vi "LVObject to JSON - JSON Array - Is Wrapped in Object.vi"() -> ()   [LabVIEW 2017, in "JSON Serializable Serializer Tests.lvlib"]
uses:
  JSON Serializable Serializer Tests.lvlib
  JSON Serializable Serializer/JSON Serializable Serializer.lvclass
  <vilib>/addons/_JKI Toolkits/Caraya/classes/Assert/Assert Equal Value_Variant.vi
  <vilib>/addons/_JKI Toolkits/Caraya/classes/Test/Test.lvclass
  <vilib>/addons/_JKI Toolkits/Caraya/classes/Assert/Assert.lvclass
  Mock JSON Serializable/Mock JSON Serializable.lvclass
panel:
  out "error out":errorcluster
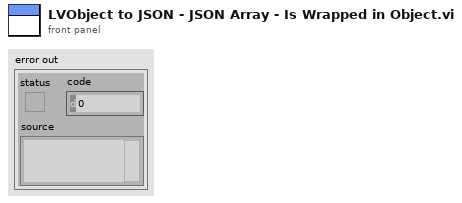
[diagram p1: front panel]
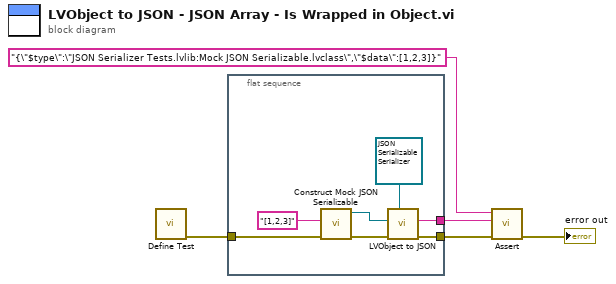
[diagram p0: block diagram]
diagram:
  n1 = call <vilib>:"Define Test.vi"() -> ("error out"=w4:errorcluster)  [unwired: 11 in]
  n2 = flat-sequence {
    tunnel: [w7] -> w5
    tunnel: w4 -> [w9]
    tunnel: [w6] -> w2
    frame #0 {
      n3 = call "Construct Mock JSON Serializable.vi"("error in (no error)"=w9, "To JSON <JSON> (\"{}\")"="[1,2,3]" ("<JSON> (\"{}\")")) -> ("error out"=w8:errorcluster, "Mock JSON Serializable"=w10:refnum<class "Mock JSON Serializable.lvclass">)  [unwired: 8 in]
      n4 = call-dynamic "LVObject to JSON.vi"("JSON Serializer in"=refnum<class "JSON Serializable Serializer.lvclass"> refnum ("JSON Serializer.lvclass"), "error in (no error)"=w8, "Object"=w10) -> ("error out"=w7:errorcluster, "<JSON>Object"=w6:string)  [unwired: 7 in]
    }
  }
  n5 = call-poly <vilib>:"Assert.vi"("error in (no error)"=w5, "Y"=w2, "X"="{\"$type\":\"JSON Serializer Tests.lvlib:Mock JSON Serializable.lvclass\",\"$data\":[1,2,3]}") -> ("error out"=→"error out":errorcluster)  [unwired: 8 in]
